vi "PSA Configure Acquisition.vi"(4 "Scale / Division (dB)":dbl=10.0, 6 "Vertical Scale (0: Linear)":i32, 7 "Enable Continuous Sweep Mode":bool, 8 "error in (no error)":errorcluster, 9 "Manual Detector Type":i32(ring) items=["Average", "Peak", "Sample", "Negative peak", "Quasi Peak", "EMI Average", "EMI Peak", "MIL Peak", "RMS"], 10 "Enable Auto Detector":bool=TRUE, 11 "VISA Refnum in":refnum<visa-resource-name>) -> (0 "error out":errorcluster, 3 "VISA Refnum out":refnum<visa-resource-name>)   [LabVIEW 2014]
uses:
  Agilent ESA PSA Series.lvlib
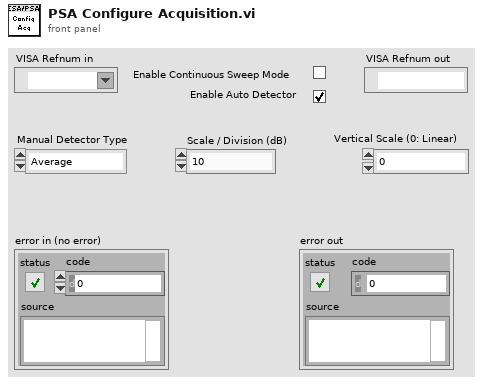
[diagram p1: front panel]
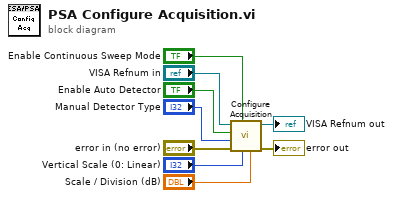
[diagram p0: block diagram]
diagram:
  n1 = call "Configure Acquisition.vi"("Scale / Division (10 dB)"="Scale / Division (dB)", "Vertical Scale (0: Linear)"="Vertical Scale (0: Linear)", "Enable Continuous Sweep Mode (F: Disable)"="Enable Continuous Sweep Mode", "error in (no error)"="error in (no error)", "Manual Detector Type (0: Average)"="Manual Detector Type", "Enable Auto Detector (T: Enable)"="Enable Auto Detector", "VISA resource name"="VISA Refnum in") -> ("error out"=→"error out":errorcluster, "VISA resource name out"=→"VISA Refnum out":refnum<visa-resource-name>)  [unwired: 3 in]
